vi "Set XTAL Frequency.vi"(8 "error in (no error)":errorcluster, 9 "Tuner Frequency":u32, 10 "RTL Frequency":u32, 11 "DeviceRefnum":u64) -> (0 "error out":errorcluster, 2 "function return":i32, 3 "DeviceRefnum Out":u64)   [LabVIEW 2014]
doc: "Set crystal oscillator frequencies used for the RTL2832 and the tuner IC."
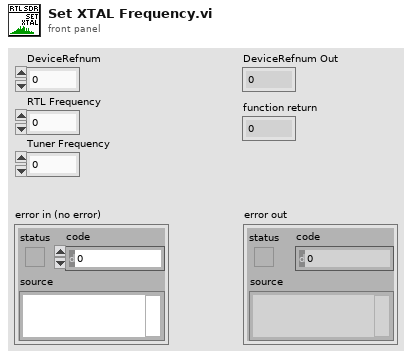
[diagram p1: front panel]
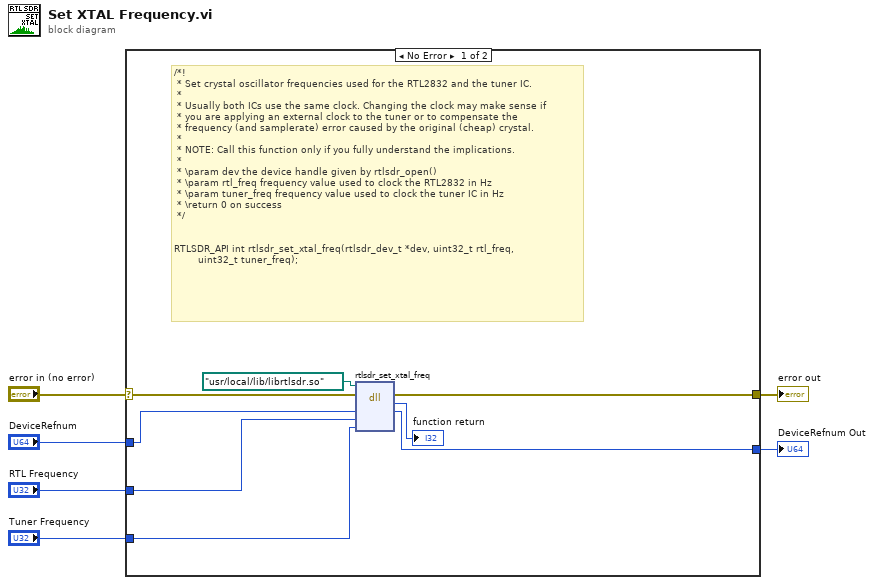
[diagram p0: block diagram]
diagram:
  n1 = case shown="No Error" "error in (no error)" {
    selector: "error in (no error)" -> [w7 w16]
    tunnel: [w13 w16] -> w6
    tunnel: "DeviceRefnum" -> [w12 w15]
    tunnel: "RTL Frequency" -> [w11 _]
    tunnel: "Tuner Frequency" -> [w10 _]
    tunnel: [w9 w15] -> w2
    frame No Error {
      # "/*!\n * Set crystal oscillator frequencies used for the RTL2832 and the tuner IC.\n *\n * Usually both ICs use the same clock. Changing the clock may make sense if\n * you are applying an external clock to the tuner or to compensate the\n * frequency (and samplerate) error caused by the original (cheap) crystal.\n *\n * NOTE: Call this function only if you fully understand the implications.\n *\n * \\param dev the device handle given by rtlsdr_open()\n * \\param rtl_freq frequency value used to clock the RTL2832 in Hz\n * \\param tuner_freq frequency value used to clock the tuner IC in Hz\n * \\return 0 on success\n */\n\n\nRTLSDR_API int rtlsdr_set_xtal_freq(rtlsdr_dev_t *dev, uint32_t rtl_freq,\n\t\t\t\t    uint32_t tuner_freq);"
      n2 = dll-call lib="C:/Program Files (x86)/National Instruments/LabVIEW 2016/user.lib/rtlsdr/rtlsdr.*" fn="rtlsdr_set_xtal_freq"(path in=path "/usr/local/lib/librtlsdr.so", error in=w7, "DeviceRefnum"=w12, "RTL Frequency"=w11, "Tuner Frequency"=w10) -> (error out=w13:errorcluster, "return type"=→"function return":i32, "DeviceRefnum"=w9:u64)  [unwired: 3 in, 1 out]
    }
    frame Error {
    }
  }
  "error out" <- w6
  "DeviceRefnum Out" <- w2
